vi "PDLM_GetDriverInfo.vi"(11 "error in (no error)":errorcluster) -> (4 "return type":i32, 6 "cName":string, 8 "cVersion":string, 10 "cDate":string, 15 "error out":errorcluster)   [LabVIEW 2019]
doc: "Gets service name, driver version and driver date"
uses:
  <userlib>/TaikoLaser/PDLM_DllPath_global.vi
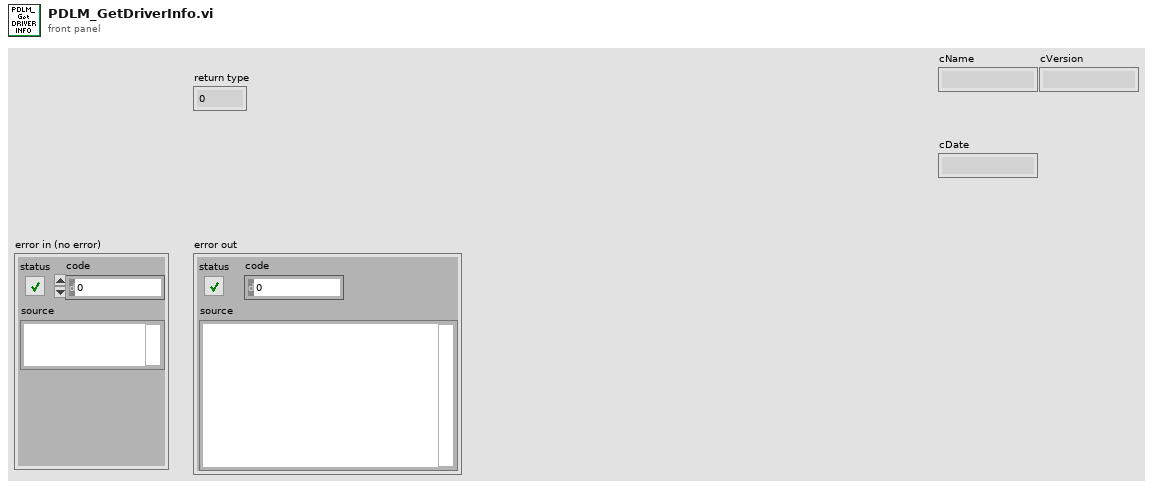
[diagram p1: front panel]
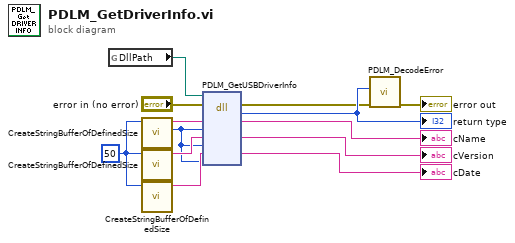
[diagram p0: block diagram]
diagram:
  w2 = 50 ("dimension size")
  n1 = global read "PDLM_DllPath_global.vi" "DllPath"() -> (w9:path)
  n2 = call <userlib>:"CreateStringBufferOfDefinedSize.vi"("size"=w2) -> ("size (out)"=w1:i32, "string"=w5:string)  [unwired: 9 in]
  n3 = call <userlib>:"CreateStringBufferOfDefinedSize.vi"("size"=w2) -> ("string"=w4:string)  [unwired: 9 in, 1 out]
  n4 = call <userlib>:"CreateStringBufferOfDefinedSize.vi"("size"=w2) -> ("string"=w3:string)  [unwired: 9 in, 1 out]
  n5 = dll-call lib="M:/_dev/progs/LabVIEW/_lib/PQ/Taiko/pdlm_lib.dll" fn="PDLM_GetUSBDriverInfo"(path in=w9, error in="error in (no error)", "cName"=w5, "uiNBuffLen"=w1, "cVersion"=w4, "uiVBuffLen"=w1, "cDate"=w3, "uiDBuffLen"=w1) -> (error out=w11:errorcluster, "return type"=w12:i32, "cName"=→"cName":string, "cVersion"=→"cVersion":string, "cDate"=→"cDate":string)  [unwired: 4 in, 1 out]
  "return type" <- w12
  n6 = call <userlib>:"PDLM_DecodeError.vi"("error in (no error)"=w11, "code"=w12) -> ("error out"=→"error out":errorcluster)  [unwired: 7 in, 2 out]
